vi "MassCompile.vi"(8 "error in (no error)":errorcluster) -> (0 "error out":errorcluster)   [LabVIEW 2020, in "CICD.lvlib"]
uses:
  CICD.lvlib
  <vilib>/Wiresmith Technology/G CLI/CLI Class/CLI.lvclass
  <vilib>/Wiresmith Technology/G CLI/Argument Parser/Option Set Class/Option Set.lvclass
  <vilib>/Wiresmith Technology/G CLI/Argument Parser/Option Class/Argument Type.ctl
  <vilib>/Wiresmith Technology/G CLI/Argument Parser/Option Class/Option.lvclass
  <vilib>/Wiresmith Technology/G CLI/Argument Parser/Option Class/Option Configuration.ctl
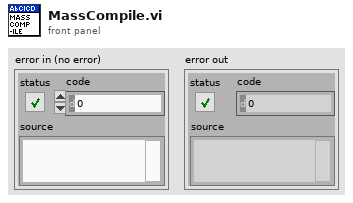
[diagram p1: front panel]
types:
  T1 = typedef "Option Parser.lvlib/Option.lvclass/Option Configuration.ctl" = cluster{"Option Type":T2, "Option Labels":string[], "Key":string, "Description":string, "Required":bool, "Default Value":string}
  T2 = typedef "Option Parser.lvlib/Option.lvclass/Argument Type.ctl" = enum16{"flag", "value"}
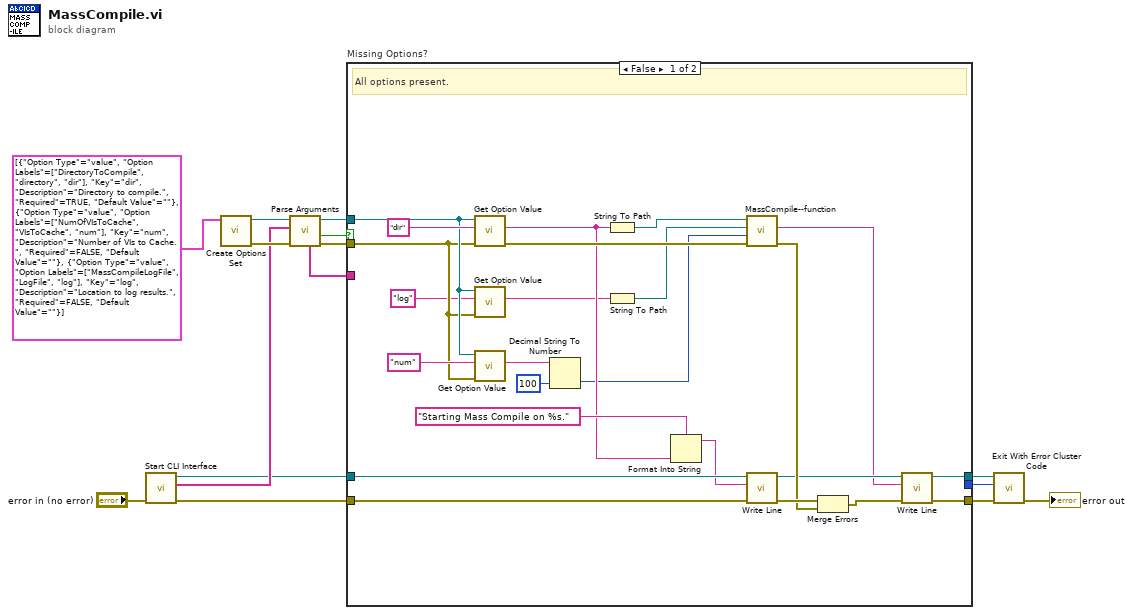
[diagram p0: block diagram]
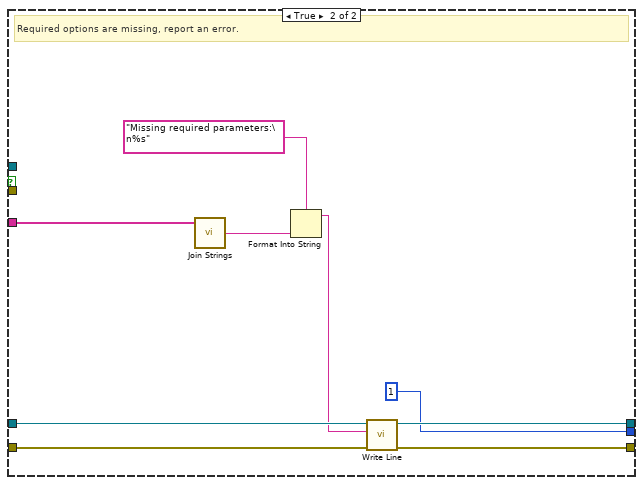
[diagram p2: hidden frame]
diagram:
  n1 = call <vilib>:"Start CLI Interface.vi"("error in (no error)"="error in (no error)") -> ("error out"=w8:errorcluster, "Custom Parameters"=w12:string[], "CLI out"=w7:refnum<class "CLI.lvclass">)  [unwired: 7 in, 1 out]
  n2 = call <vilib>:"Create Options Set.vi"("Options"=T1[] [{"Option Type"=enum."value", "Option Labels"=["DirectoryToCompile", "directory", "dir"], "Key"="dir", "Description"="Directory to compile.", "Required"=TRUE, "Default Value"=""}, {"Option Type"=enum."value", "Option Labels"=["NumOfVIsToCache", "VIsToCache", "num"], "Key"="num", "Description"="Number of VIs to Cache.", "Required"=FALSE, "Default Value"=""}, {"Option Type"=enum."value", "Option Labels"=["MassCompileLogFile", "LogFile", "log"], "Key"="log", "Description"="Location to log results.", "Required"=FALSE, "Default Value"=""}]) -> ("error out"=w13:errorcluster, "Option Set out"=w14:refnum<class "Option Set.lvclass">)  [unwired: 9 in]
  n3 = call <vilib>:"Parse Arguments.vi"("error in (no error)"=w13, "Arguments"=w12, "Option Set in"=w14) -> ("error out"=w10:errorcluster, "Missing Options"=w11:bool, "Option Set out"=w2:refnum<class "Option Set.lvclass">, "Missing Option Keys"=w9:string[])  [unwired: 5 in]
  n4 = case "Missing Options?" shown="False" w11 {
    tunnel: w10 -> [w24 _]
    tunnel: w9 -> [_ w46]
    tunnel: w8 -> [w39 w45]
    tunnel: w7 -> [w36 w44]
    tunnel: [w19 w42] -> w6
    tunnel: [w17 w41] -> w4
    tunnel: [_ 1 ("No Error Code (0)")] -> w3
    tunnel: w2 -> [w25 _]
    frame False {
      # "All options present."
      n5 = call <vilib>:"Get Option Value.vi"("error in (no error)"=w24, "Option Key"="dir", "Option Set in"=w25) -> ("error out"=w32:errorcluster, "Value"=w29:string)  [unwired: 5 in, 2 out]
      n6 = call <vilib>:"Get Option Value.vi"("error in (no error)"=w24, "Option Key"="log", "Option Set in"=w25) -> ("Value"=w22:string)  [unwired: 5 in, 3 out]
      n7 = call <vilib>:"Get Option Value.vi"("error in (no error)"=w24, "Option Key"="num", "Option Set in"=w25) -> ("Value"=w27:string)  [unwired: 5 in, 3 out]
      n8 = Decimal String To Number(string=w27, default (0L)=u32 100 ("default (0 I32)")) -> (number=w20:u32)  [unwired: 1 in, 1 out]
      n9 = String To Path(string=w29) -> (path=w28:path)
      n10 = String To Path(string=w22) -> (path=w21:path)
      n11 = Format Into String(format string="Starting Mass Compile on %s.", w29) -> (resulting string=w33:string)  [unwired: 2 in, 1 out]
      n12 = call "MassCompile--function.vi"("error in"=w32, "Number of VIs to Cache"=w20, "Mass Compile Log File"=w21, "Directory to Compile"=w28) -> ("error out"=w31:errorcluster, "log text"=w16:string)  [unwired: 6 in]
      n13 = call <vilib>:"Write Line.vi"("error in (no error)"=w39, "Text to Write"=w33, "CLI in"=w36) -> ("error out"=w37:errorcluster, "CLI out"=w18:refnum<class "CLI.lvclass">)  [unwired: 7 in]
      n14 = Merge Errors(w37, w31) -> (w35:errorcluster)
      n15 = call <vilib>:"Write Line.vi"("error in (no error)"=w35, "Text to Write"=w16, "CLI in"=w18) -> ("error out"=w19:errorcluster, "CLI out"=w17:refnum<class "CLI.lvclass">)  [unwired: 7 in]
    }
    frame True {
      # "Required options are missing, report an error."
      n16 = call <vilib>:"Join Strings.vi"("Strings In"=w46) -> ("String"=w47:string)  [unwired: 2 in]
      n17 = Format Into String(format string="Missing required parameters:\n%s" ("Text to Write"), w47) -> (resulting string=w43:string)  [unwired: 2 in, 1 out]
      n18 = call <vilib>:"Write Line.vi"("error in (no error)"=w45, "Text to Write"=w43, "CLI in"=w44) -> ("error out"=w42:errorcluster, "CLI out"=w41:refnum<class "CLI.lvclass">)  [unwired: 7 in]
    }
  }
  n19 = call <vilib>:"Exit With Error Cluster Code.vi"("error in (no error)"=w6, "No Error Code (0)"=w3, "CLI in"=w4) -> ("error out"=→"error out":errorcluster)  [unwired: 8 in]
